vi "Get ID from Position.vi"(10 "Row":i32, 11 "Column":i32) -> (3 "Position ID":T1)   [LabVIEW 2017, in "AntFarm_MB.lvclass"]
uses:
  AntFarm_MB.lvclass
  TypeDefs/ENUM_Position ID.ctl
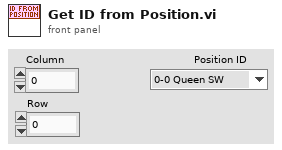
[diagram p1: front panel]
types:
  T1 = typedef "ENUM_Position ID.ctl" = enum16{"0-0 Queen SW", "0-1 Path E", "0-2 Queen NW", "0-3 Path W", "1-0 Path S", "1-1 Larva SW", "1-2 Path N", "1-3 Larva NW", "2-0 Queen SE", "2-1 Path W", "2-2 Queen NE", "2-3 Path E", "3-0 Path N", "3-1 Larva SE", "3-2 Path S", "3-3 Larva NE"}
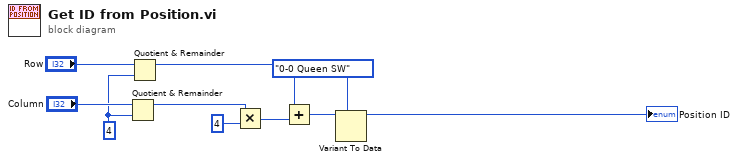
[diagram p0: block diagram]
diagram:
  w1 = 4 ("y")
  n1 = Quotient & Remainder(x="Column", y=w1) -> (x-y*floor(x/y)=w4:i32)  [unwired: 1 out]
  n2 = Quotient & Remainder(x="Row", y=w1) -> (x-y*floor(x/y)=w2:i32)  [unwired: 1 out]
  n3 = Multiply(x=w4, y=4) -> (x*y=w9:i32)
  n4 = Add(x=w2, y=w9) -> (x+y=w6:i32)
  n5 = Variant To Data(type=ENUM_Position_ID."0-0 Queen SW" ("Position ID"), Variant=w6) -> (data=→"Position ID":T1)  [unwired: 1 in, 1 out]
